vi "LockinDAQ.getAOChannels.vi"(8 "error in (no error)":errorcluster, 10 "Channels: AO":T1={"Ch"=[], "Amp (V)"=[0.01, 0.0, 0.0, 0.0, 0.0, 0.0, 0.0, 0.0], "DC (V)"=[0.0, 0.0, 0.0, 0.0, 0.0, 0.0, 0.0, 0.0], "f (Hz)"=[0.0, 0.0, 0.0, 0.0, 0.0, 0.0, 0.0, 0.0], "Phase (°)"=[13.1, 13.0, 13.0, 13.0, 13.0, 13.0, 13.0, 13.0], "Function"=[enum."Sine", enum."Sine", enum."Sine", enum."Sine", enum."Sine", enum."Sine", enum."Sine", enum."Sine"], "Sweep?"=[FALSE, FALSE, FALSE, FALSE, FALSE, FALSE, FALSE, FALSE]} {"f (Hz)" min=0.001 max=10000.0; "DC (V)" format="%.3p"; "Amp (V)" format="%.3p"}, 11 "LockinDAQ":refnum<class "LockinDAQ.lvclass">) -> (0 "error out":errorcluster, 3 "LockinDAQ out":refnum<class "LockinDAQ.lvclass">)   [LabVIEW 2016, in "LockinDAQ.lvclass"]
doc: "---------------------------------------------------------------\nJKI State Machine Objects™\nhttp://jki.net/state-machine-objects/\nCopyright (C) 2005-2015, JKI <info@jki.net>\nALL RIGHTS RESERVEDJKI State Machine Objects (SMO) 1.0.0.4\nJKI - JKI\nCopyright (c) 2015, JKI"
uses:
  LockinDAQ.lvclass
  Typedefs/AO-cluster.ctl
  Typedefs/Function-enum.ctl
  LockinDAQ.lvclass/LockinDAQ.ctl
panel:
  # "For instructions on how to use the JKI State Machine Objects, examples and video tutorials, visit:\nhttp://jki.net/state-machine-objects/\n\nJKI State Machine Objects™\nhttp://jki.net/state-machine-objects/\nCopyright (C) 2005-2015, JKI <info@jki.net>\nALL RIGHTS RESERVED"
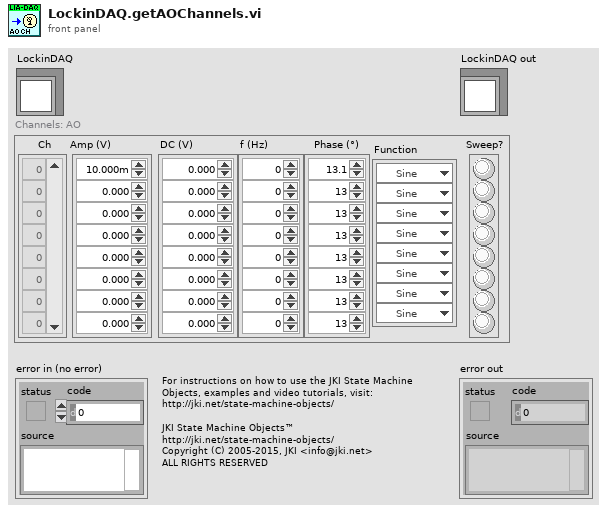
[diagram p1: front panel]
types:
  T1 = typedef "LockinDAQ.lvclass/AO-cluster.ctl" = cluster{"Ch":i32[], "Amp (V)":dbl[], "DC (V)":dbl[], "f (Hz)":dbl[], "Phase (°)":dbl[], "Function":T2[], "Sweep?":bool[]}
  T2 = typedef "LockinDAQ.lvclass/Function-enum.ctl" = enum16{"Sine", "Triangle", "Square", "Sawtooth"}
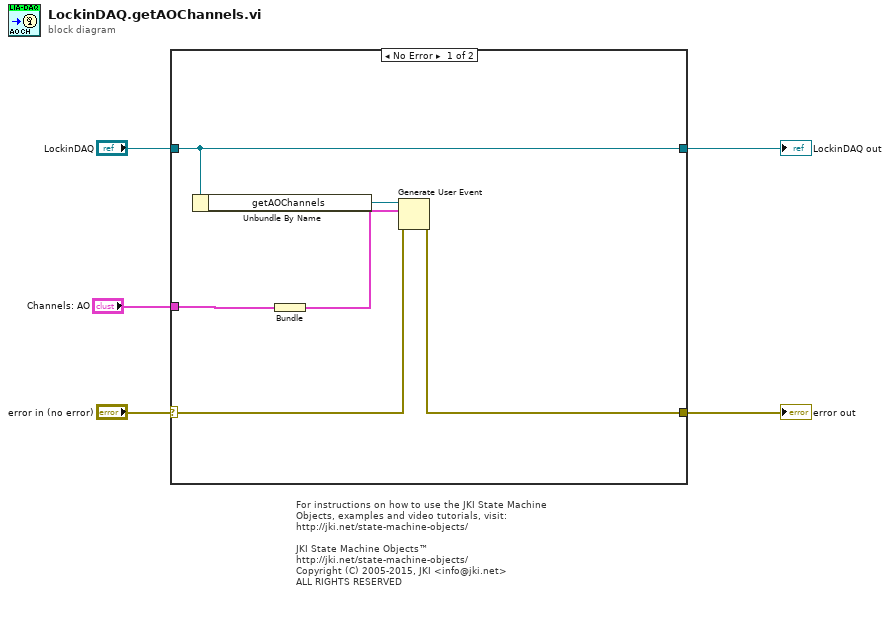
[diagram p0: block diagram]
diagram:
  # "For instructions on how to use the JKI State Machine Objects, examples and video tutorials, visit:\nhttp://jki.net/state-machine-objects/\n\nJKI State Machine Objects™\nhttp://jki.net/state-machine-objects/\nCopyright (C) 2005-2015, JKI <info@jki.net>\nALL RIGHTS RESERVED"
  n1 = case shown="No Error" "error in (no error)" {
    selector: "error in (no error)" -> [w11 w13]
    tunnel: [w9 w13] -> w4
    tunnel: [w8 w12] -> w5
    tunnel: "LockinDAQ" -> [w8 w12]
    tunnel: "Channels: AO" -> [w7 _]
    frame No Error {
      n2 = Unbundle By Name(w8) -> ("getAOChannels"=w10:refnum<user-event>)
      n3 = Bundle("Channels: AO"=w7) -> (w6:cluster{"Channels: AO":T1})  [unwired: 1 in]
      n4 = Generate User Event(user event=w10, event data cluster=w6, error in=w11) -> (error out=w9:errorcluster)  [unwired: 1 in, 1 out]
    }
    frame Error {
    }
  }
  "error out" <- w4
  "LockinDAQ out" <- w5
